vi "SubVI_02.vi"(10 "string array":string[](array[string]), 11 "String":string) -> (1 "Last":i32, 2 "First":i32, 3 "Array":T1(array[cluster]))   [LabVIEW 2023]
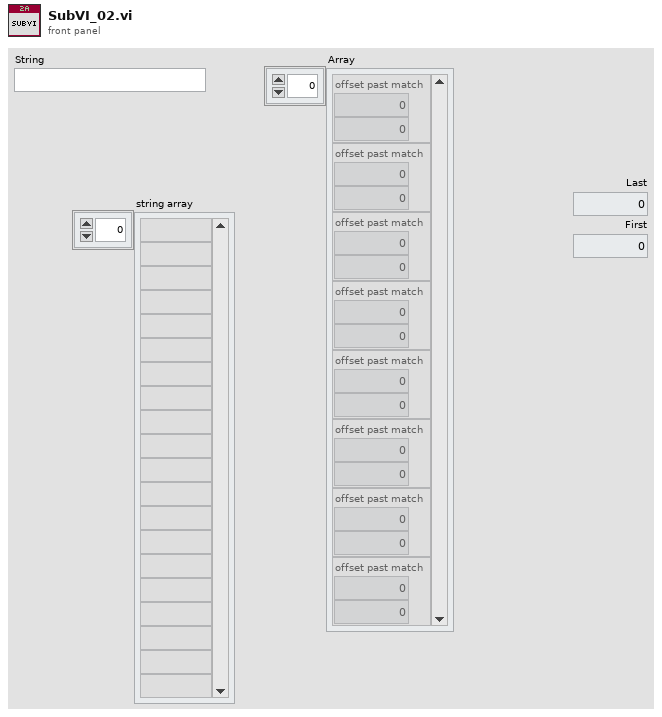
[diagram p1: front panel]
types:
  T1 = cluster{"offset past match":i32, "Numeric":i32}[]
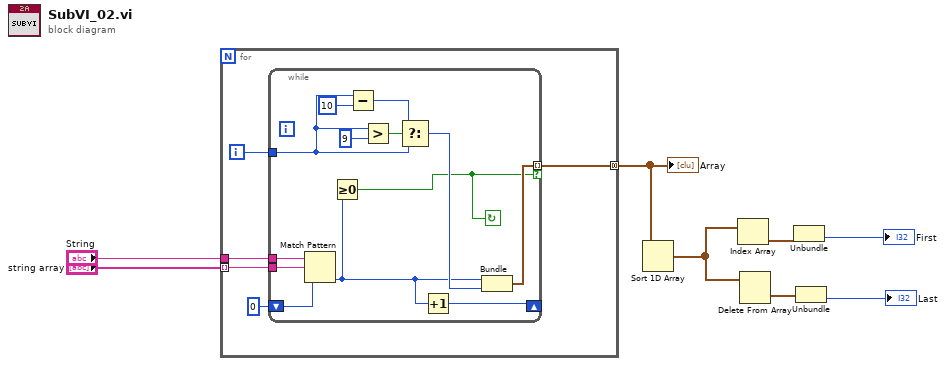
[diagram p0: block diagram]
diagram:
  n1 = for {
    tunnel: "string array" -> [w13] mode=indexing
    tunnel: [w12] -> w5 mode=concatenating
    tunnel: "String" -> [w11]
    i -> [w9]
    n2 = while {
      tunnel: w11 -> [w26]
      tunnel: w13 -> [w25]
      tunnel: [w19] -> w12 mode=indexing if=w18
      shift-right: [w16] -> _
      shift-left: 0 -> [w15]
      tunnel: w9 -> [w14]
      stop <- w18 continue-if-true
      n3 = Match Pattern(string=w26, regular expression=w25, offset (0)=w15) -> (offset past match=w17:i32)  [unwired: 3 out]
      n4 = Greater Or Equal To 0?(x=w17) -> (x >= 0?=w18:bool)
      n5 = Subtract(x=w14, y=10) -> (x-y=w21:i32)
      n6 = Greater?(x=w14, y=9) -> (0:w23:bool)
      n7 = Select(t=w21, s=w23, f=w14) -> (s? t:f=w20:i32)
      n8 = Increment(x=w17) -> (x+1=w16:i32)
      n9 = Bundle("offset past match"=w17, w20) -> (w19:cluster{"offset past match":i32, i32})  [unwired: 1 in]
    }
  }
  "Array" <- w5
  n10 = Sort 1D Array(array=w5) -> (sorted array=w6:cluster{"offset past match":i32, i32}[])
  n11 = Index Array(array=w6) -> (element=w4:cluster{"offset past match":i32, i32})  [unwired: 1 in]
  n12 = Delete From Array(array=w6) -> (deleted portion=w3:cluster{"offset past match":i32, i32})  [unwired: 2 in, 1 out]
  n13 = Unbundle(w4) -> (→"First":i32)  [unwired: 1 out]
  n14 = Unbundle(w3) -> (→"Last":i32)  [unwired: 1 out]
